vi "Read Image Data.vi"(8 "Input Index":u32, 10 "PatchHeader":T1, 11 "Patch DATA IN":u8[](array[numeric])) -> (0 "Output Index":u32, 1 "Mask OUT":u8[](array[numeric]), 2 "Image OUT":u8[][](array[numeric]), 3 "Patch DATA OUT":u8[](array[numeric]))   [LabVIEW 2017]
uses:
  PatchHeader.ctl
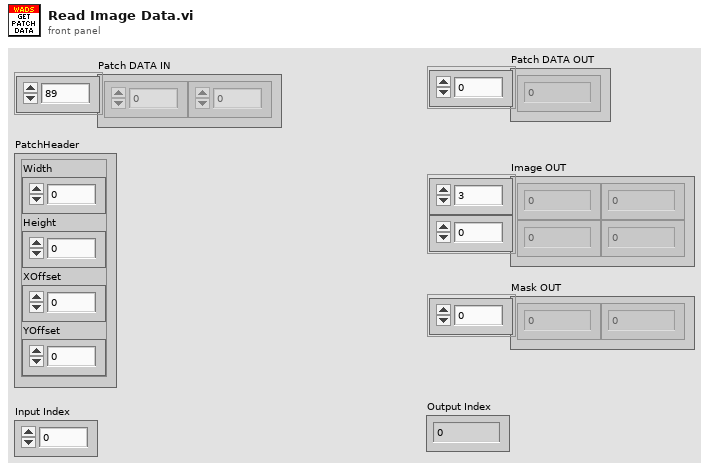
[diagram p1: front panel]
types:
  T1 = typedef "PatchHeader.ctl" = cluster{"Width":u16, "Height":u16, "XOffset":i16, "YOffset":i16}
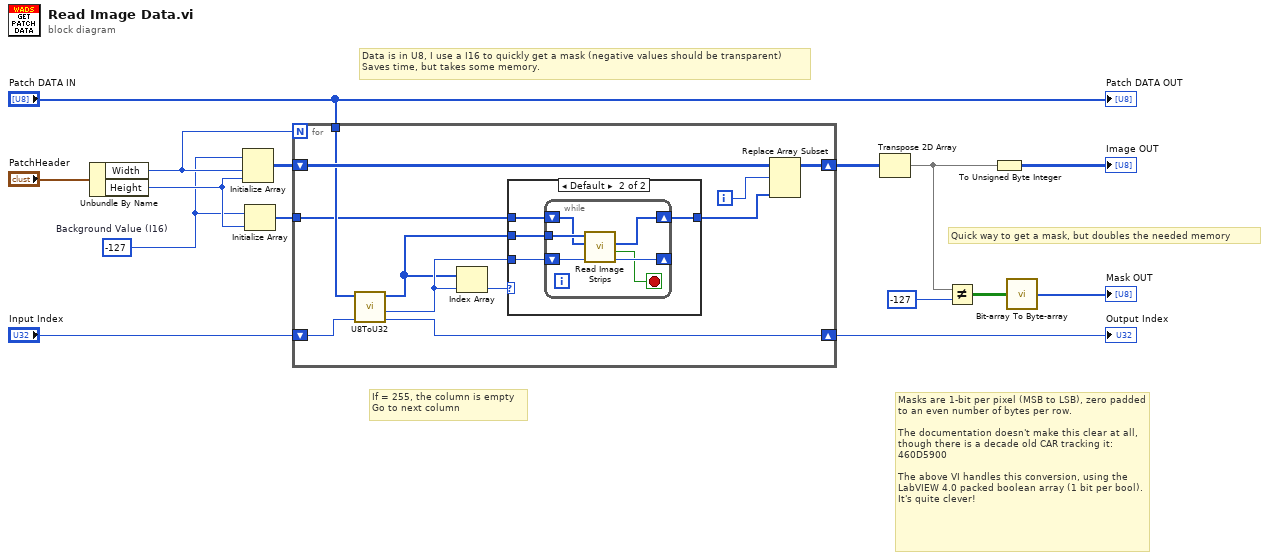
[diagram p0: block diagram]
diagram:
  w7 = i16 -127  # Background Value (I16)
  # "Masks are 1-bit per pixel (MSB to LSB), zero padded to an even number of bytes per row.\n\nThe documentation doesn't make this clear at all, though there is a decade old CAR tracking it: 460D5900\n\nThe above VI handles this conversion, using the LabVIEW 4.0 packed boolean array (1 bit per bool). It's quite clever!"
  # "If = 255, the column is empty\nGo to next column"
  # "Data is in U8, I use a I16 to quickly get a mask (negative values should be transparent)\nSaves time, but takes some memory."
  # "Quick way to get a mask, but doubles the needed memory"
  n1 = Unbundle By Name("PatchHeader") -> ("Width"=w10:u16, "Height"=w11:u16)
  n2 = Initialize Array(w7, w10, w11) -> (w14:i16[][])
  n3 = Initialize Array(w7, w11) -> (w13:i16[])
  n4 = for {
    N: w10 -> [_]
    tunnel: w13 -> [w19]
    tunnel: "Patch DATA IN" -> [w24]
    shift-right: [w25] -> w6
    shift-left: w14 -> [w26]
    shift-right: [w22] -> w8
    shift-left: "Input Index" -> [w23]
    i -> [w21]
    n5 = call "U8ToU32.vi"("Index"=w23, "Input U8 Array"=w24) -> ("Index+4"=w22:u32, "Output U32"=w18:u32, "Output U8 Array"=w17:u8[])  [unwired: 3 in]
    n6 = Index Array(array=w17, index=w18) -> (element=w16:u8)
    n7 = case shown="Default" w16 {
      tunnel: w17 -> [_ w31]
      tunnel: [w27 w30] -> w20
      tunnel: w19 -> [w27 w29]
      tunnel: w18 -> [_ w28]
      frame 255 {
      }
      frame Default {
        n8 = while {
          tunnel: w31 -> [w37]
          shift-right: [w33] -> _
          shift-left: w28 -> [w36]
          shift-right: [w34] -> w30
          shift-left: w29 -> [w35]
          stop <- w32 stop-if-true
          n9 = call "Read Image Strips.vi"("First Strip"=w36, "Column IN"=w35, "DATA IN"=w37) -> ("Next Strip"=w33:u32, "Enf of Column?"=w32:bool, "Column OUT"=w34:i16[])  [unwired: 6 in]
        }
      }
    }
    n10 = Replace Array Subset(array=w26, new element=w20, index (row)=w21) -> (w25:i16[][])  [unwired: 1 in]
  }
  "Output Index" <- w8
  n11 = Transpose 2D Array(2D array=w6) -> (transposed array=w5:i16[][])
  n12 = Not Equal?(x=w5, y=i16 -127 ("Index")) -> (x != y?=w2:bool[][])
  n13 = To Unsigned Byte Integer(number=w5) -> (unsigned 8bit integer=→"Image OUT":u8[][])
  n14 = call <vilib>:"Bit-array To Byte-array.vi"("bit array"=w2) -> ("byte array"=→"Mask OUT":u8[])
  "Patch DATA OUT" <- "Patch DATA IN"
